vi "Meter Example_EVS.vi"() -> ()   [LabVIEW 2017]
doc: "This example shows how to use the NI Vision meter reading VIs to read the position of a needle. These VIs are useful in many applications such as the calibration of speedometers and gauges in industries such as the automotive industry."
uses:
  <vilib>/vision/NI_Vision_Development_Module.lvlib
panel:
  out "Meter":dbl(knob)=41.86465883402845 scale=0.0..100.0
  out "Image":T1(plugin-control)
  in  "Delay":i32(slide)=738 max=3000 scale=0.0..1000.0
  in  "stop":bool
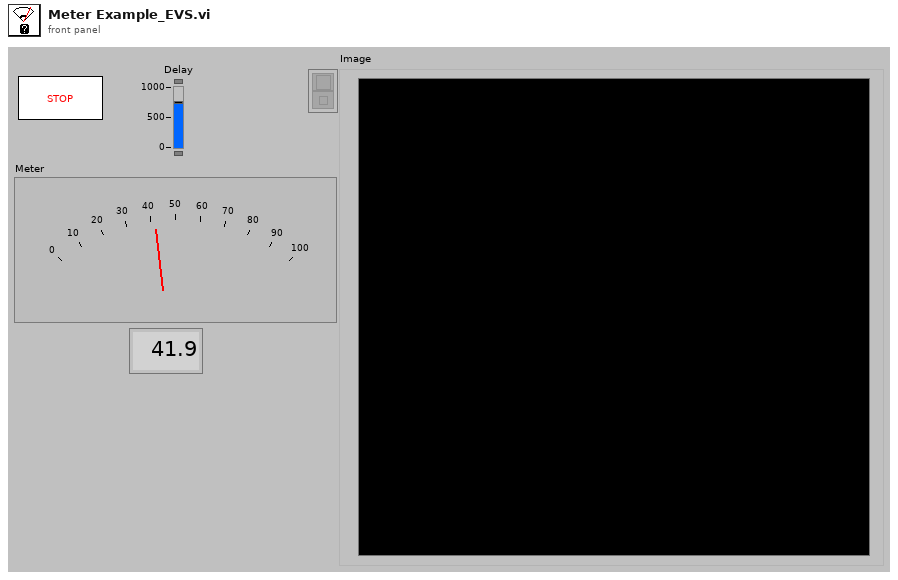
[diagram p1: front panel]
types:
  T1 = typedef "IMAQ Image.ctl" = refnum<image>
  T2 = cluster{"Global Rectangle":i32[], "Contours":cluster{"Contour Type":u32, "ROI Type":u32, "Points":i32[]}[]}[]
  T3 = typedef "ROI Descriptor" = cluster{"Global Rectangle":i32[], "Contours":cluster{"ID":enum32{"External", "Internal"}, "Type":u32, "Coordinates":i32[]}[]}
  T4 = cluster{"[0]":sgl, "[1]":sgl, "[2]":sgl, "[3]":sgl}
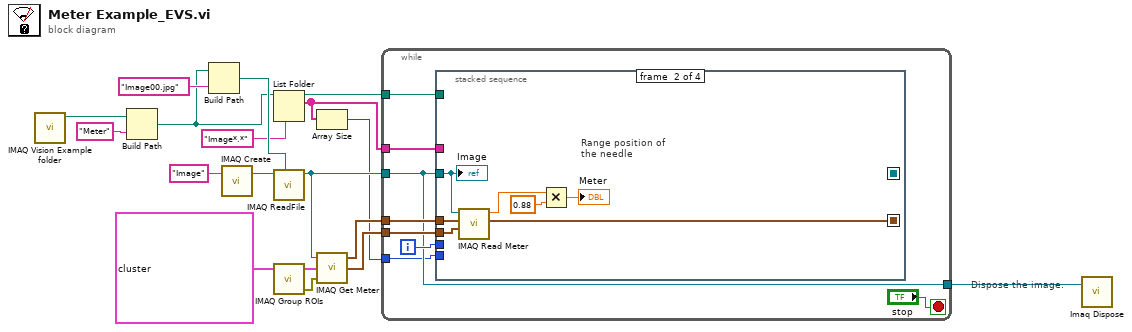
[diagram p0: block diagram]
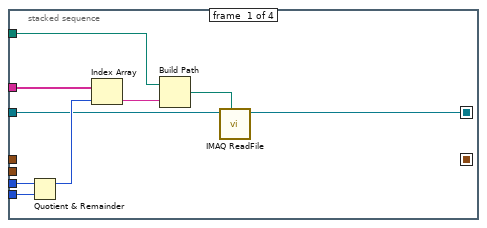
[diagram p2: hidden frame]
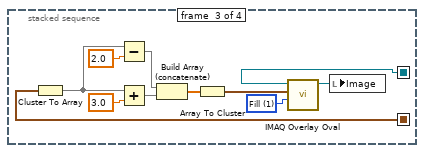
[diagram p3: hidden frame]
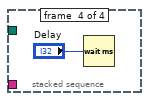
[diagram p4: hidden frame]
diagram:
  # "Dispose the image."
  n1 = call "IMAQ Vision Example folder.vi"() -> ("Example Image Path"=w11:path)  [unwired: 11 in]
  n2 = Build Path(base path=w11, name or relative path="Meter") -> (appended path=w1:path)
  n3 = Build Path(base path=w1, name or relative path="Image00.jpg") -> (appended path=w12:path)
  n4 = call "IMAQ Create"("Image Name"="Image") -> ("New Image"=w13:T1)  [unwired: 3 in, 2 out]
  n5 = List Folder(path=w1, pattern="Image*.*") -> (path out=w3:path, filenames=w4:string[])  [unwired: 1 in, 3 out]
  n6 = call "IMAQ ReadFile"("File Path"=w12, "Image"=w13) -> ("Image Out"=w7:T1)  [unwired: 3 in, 6 out]
  n7 = call "IMAQ Group ROIs"("ROI Descriptors"=T2 [{"Global Rectangle"=[52, 75, 124, 165], "Contours"=[{"Contour Type"=0, "ROI Type"=2, "Points"=[52, 75, 123, 164]}]}, {"Global Rectangle"=[133, 62, 191, 165], "Contours"=[{"Contour Type"=0, "ROI Type"=2, "Points"=[190, 62, 133, 164]}]}] ("appended array")) -> ("error out"=w8:errorcluster, "ROI Descriptor out"=w9:T3)  [unwired: 1 in, 2 out]
  n8 = Array Size(array=w4) -> (size(s)=w2:i32)
  n9 = call "IMAQ Get Meter"("Image"=w7, "ROI Descriptor"=w9, "error in (no error)"=w8) -> ("Needle Base"=w17:cluster{"X":sgl, "Y":sgl}, "Points Arc"=w18:cluster{"X":sgl, "Y":sgl}[])  [unwired: 5 out]
  n10 = while {
    tunnel: w17 -> [w24]
    tunnel: w18 -> [w25]
    tunnel: w7 -> [w22]
    tunnel: [w22] -> w6
    tunnel: w4 -> [w21]
    tunnel: w3 -> [w20]
    tunnel: w2 -> [w19]
    i -> [w23]
    stop <- "stop" stop-if-true
    n11 = stacked-sequence {
      seq-local: [w32 _ _ _] -> [_ _ w45 _]
      seq-local: [_ w38 _ _] -> [_ _ w53 _]
      tunnel: w25 -> [_ w42 _ _]
      tunnel: w24 -> [_ w41 _ _]
      tunnel: w23 -> [w30 _ _ _]
      tunnel: w22 -> [w31 w37 _ _]
      tunnel: w21 -> [w29 _ _ _]
      tunnel: w20 -> [w28 _ _ _]
      tunnel: w19 -> [w27 _ _ _]
      frame #0 {
        n12 = Quotient & Remainder(x=w30, y=w27) -> (x-y*floor(x/y)=w35:i32)  [unwired: 1 out]
        n13 = Index Array(array=w29, index=w35) -> (element=w34:string)
        n14 = Build Path(base path=w28, name or relative path=w34) -> (appended path=w33:path)
        n15 = call "IMAQ ReadFile"("File Path"=w33, "Image"=w31) -> ("Image Out"=w32:T1)  [unwired: 3 in, 6 out]
      }
      frame #1 {
        # "Range position of \nthe needle"
        n16 = call "IMAQ Read Meter"("Arc Points"=w42, "Needle Base"=w41, "Image"=w37) -> ("Point"=w38:cluster{"X":sgl, "Y":sgl}, "Percentage of scale"=w40:dbl)  [unwired: 2 in, 5 out]
        n17 = Multiply(x=w40, y=0.88) -> (x*y=→"Meter":dbl)
        "Image" <- w37
      }
      frame #2 {
        w44 = u32 1 items=["Frame", "Fill"] ("Drawing Mode (Frame)")
        n18 = Cluster To Array(cluster=w53) -> (array=w52:sgl[])
        n19 = Subtract(x=w52, y=sgl 2.0) -> (x-y=w50:sgl[])
        n20 = Add(x=w52, y=sgl 3.0) -> (x+y=w49:sgl[])
        n21 = Build Array (concatenate)(w50, w49) -> (w47:sgl[])
        n22 = Array To Cluster(array=w47) -> (cluster=w46:T4)
        n23 = call "IMAQ Overlay Oval"("Drawing Mode (Frame)"=w44, "Bounding Rectangle"=w46, "Image"=w45) -> ("Image Out"=w43:T1)  [unwired: 3 in, 5 out]
        n24 = local write "Image"(w43) -> ()
      }
      frame #3 {
        n25 = Wait (ms)(milliseconds to wait="Delay") -> ()  [unwired: 1 out]
      }
    }
  }
  n26 = call "Imaq Dispose"("Image"=w6) -> ()  [unwired: 2 in, 4 out]
